vi "DSF Configuration File to Cluster.vi"(8 "error in (no error)":errorcluster, 11 "dsf configuration file path":path) -> (0 "error out":errorcluster, 2 "framework configuration out":T1, 3 "dsf configuration file path dup":path)   [LabVIEW 2017, in "DSF Core.lvlib"]
uses:
  DSF Core.lvlib
  Configuration Session.lvclass
  Read Settings.vi
  Read Plugin.vi
  Typedefs/DSF Engine Channel Configuration.ctl
  Typedefs/DSF Engine Transfer Configuration.ctl
  Typedefs/DSF Engine Transfer Group Configuration.ctl
  Typedefs/DSF Engine Plugin Configuration.ctl
  Typedefs/DSF Engine Framework Configuration.ctl
  Typedefs/DSF Settings Info.ctl
  Typedefs/DSF Timing Info.ctl
  Typedefs/DSF Byte Order.ctl
  Typedefs/DSF Data Type.ctl
  Typedefs/DSF Direction.ctl
  Read All Plugin IDs.vi
  Read Group.vi
  Typedefs/DSF Engine Plugin Thread Configuration.ctl
  Typedefs/DSF Timeout Behavior.ctl
  Read Channel.vi
  Read Transfer.vi
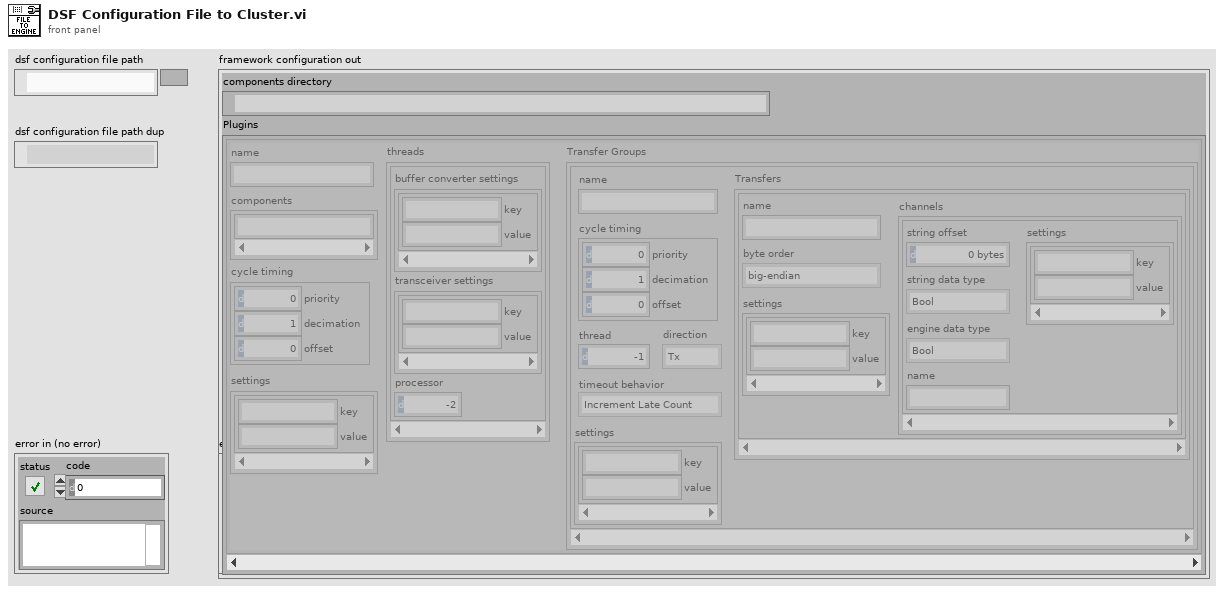
[diagram p1: front panel]
types:
  T1 = typedef "DSF Core.lvlib/DSF Engine Framework Configuration.ctl" = cluster{"components directory":path, "Plugins":T2[]}
  T2 = typedef "DSF Core.lvlib/DSF Engine Plugin Configuration.ctl" = cluster{"name":string, "components":string[], "cycle timing":T3, "threads":T4[], "Transfer Groups":T6[], "settings":T5}
  T3 = typedef "DSF Core.lvlib/DSF Timing Info.ctl" = cluster{"priority":u64, "decimation":u64, "offset":u64}
  T4 = typedef "DSF Core.lvlib/DSF Engine Plugin Thread Configuration.ctl" = cluster{"buffer converter settings":T5, "transceiver settings":T5, "processor":i32}
  T5 = typedef "DSF Core.lvlib/DSF Settings Info.ctl" = cluster{"key":string, "value":string}[]
  T6 = typedef "DSF Core.lvlib/DSF Engine Transfer Group Configuration.ctl" = cluster{"name":string, "direction":T7, "cycle timing":T3, "thread":i32, "settings":T5, "Transfers":T8[], "timeout behavior":T12}
  T7 = typedef "DSF Core.lvlib/DSF Direction.ctl" = enum8{"Tx", "Rx"}
  T8 = typedef "DSF Core.lvlib/DSF Engine Transfer Configuration.ctl" = cluster{"name":string, "byte order":T9, "settings":T5, "channels":T10[]}
  T9 = typedef "DSF Core.lvlib/DSF Byte Order.ctl" = enum8{"big-endian", "little-endian"}
  T10 = typedef "DSF Core.lvlib/DSF Engine Channel Configuration.ctl" = cluster{"string offset":u64, "string data type":T11, "engine data type":T11, "name":string, "settings":T5}
  T11 = typedef "DSF Core.lvlib/DSF Data Type.ctl" = enum8{"Bool", "SGL", "DBL", "I8", "I16", "I32", "I64", "U8", "U16", "U32", "U64"}
  T12 = typedef "DSF Core.lvlib/DSF Timeout Behavior.ctl" = enum8{"Increment Late Count", "Throw Error"}
  T13 = typedef "DSF Core.lvlib/DSF Plugin Info.ctl" = cluster{"components":string[], "timing":T3, "group ids":string[], "settings id":string, "threads":T4[]}
  T14 = typedef "DSF Core.lvlib/DSF Group Info.ctl" = cluster{"direction":T7, "timing":T3, "transfer ids":string[], "settings id":string, "thread":i32, "timeout behavior":T12}
  T15 = typedef "DSF Core.lvlib/DSF Transfer Info.ctl" = cluster{"byte order":T9, "channel ids":string[], "settings id":string}
  T16 = typedef "DSF Core.lvlib/DSF Channel Info.ctl" = cluster{"string buffer offset":u64, "string data type":T11, "engine data type":T11, "settings id":string}
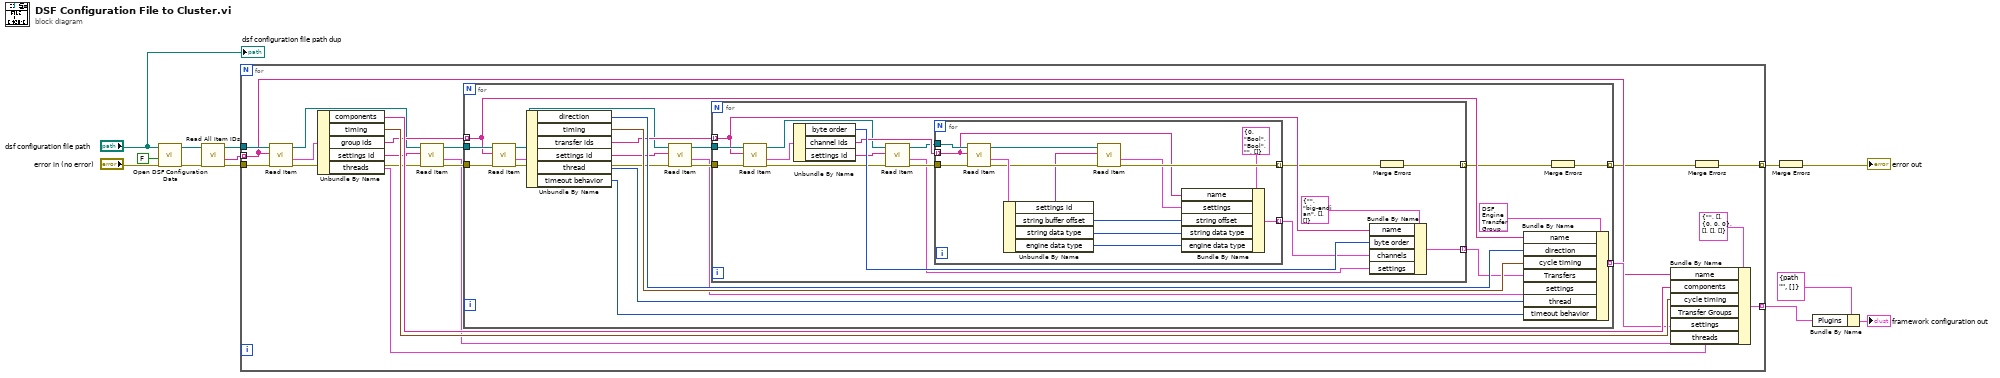
[diagram p0: block diagram]
diagram:
  n1 = call "Open DSF Configuration Data.vi"("error in (no error)"="error in (no error)", "replace if found? (F)"=FALSE ("create file if necessary (T)"), "dsf configuration file path"="dsf configuration file path") -> ("error out"=w4:errorcluster, "Configuration Session"=w5:refnum<class "Configuration Session.lvclass">)  [unwired: 4 in, 3 out]
  n2 = call-poly "Read All Item IDs.vi"("error in (no error)"=w4, "Configuration Session in"=w5) -> ("error out"=w10:errorcluster, "Plugin IDs"=w12:string[], "Configuration Session out"=w11:refnum<class "Configuration Session.lvclass">)  [unwired: 7 in]
  n3 = for {
    tunnel: w12 -> [w24] mode=indexing
    tunnel: w11 -> [w31]
    tunnel: [w27] -> w6 mode=indexing
    tunnel: w10 -> [w19]
    tunnel: [w16] -> w9 mode=indexing
    n4 = call-poly "Read Item.vi"("error in (no error)"=w19, "Plugin ID"=w24, "Configuration Session in"=w31) -> ("error out"=w20:errorcluster, "value"=w30:T13, "Configuration Session out"=w23:refnum<class "Configuration Session.lvclass">)  [unwired: 5 in, 1 out]
    n5 = Unbundle By Name(w30) -> ("components"=w29:string[], "timing"=w28:T3, "group ids"=w26:string[], "settings id"=w21:string, "threads"=w15:T4[])
    n6 = call-poly "Read Item.vi"("error in (no error)"=w20, "Settings ID"=w21, "Configuration Session in"=w23) -> ("error out"=w18:errorcluster, "value"=w14:T5, "Configuration Session out"=w22:refnum<class "Configuration Session.lvclass">)  [unwired: 5 in, 1 out]
    n7 = for {
      tunnel: w22 -> [w52]
      tunnel: w26 -> [w49] mode=indexing
      tunnel: [w46] -> w25 mode=indexing
      tunnel: w18 -> [w43]
      tunnel: [w35] -> w17 mode=indexing
      n8 = call-poly "Read Item.vi"("error in (no error)"=w43, "Group ID"=w49, "Configuration Session in"=w52) -> ("error out"=w39:errorcluster, "value"=w50:T14, "Configuration Session out"=w42:refnum<class "Configuration Session.lvclass">)  [unwired: 5 in, 1 out]
      n9 = Unbundle By Name(w50) -> ("direction"=w48:T7, "timing"=w47:T3, "transfer ids"=w45:string[], "settings id"=w40:string, "thread"=w34:i32, "timeout behavior"=w33:T12)
      n10 = call-poly "Read Item.vi"("error in (no error)"=w39, "Settings ID"=w40, "Configuration Session in"=w42) -> ("error out"=w38:errorcluster, "value"=w37:T5, "Configuration Session out"=w41:refnum<class "Configuration Session.lvclass">)  [unwired: 5 in, 1 out]
      n11 = for {
        tunnel: w45 -> [w62] mode=indexing
        tunnel: w41 -> [w69]
        tunnel: [w66] -> w44 mode=indexing
        tunnel: w38 -> [w61]
        tunnel: [w54] -> w36 mode=indexing
        n12 = call-poly "Read Item.vi"("error in (no error)"=w61, "Transfer ID"=w62, "Configuration Session in"=w69) -> ("error out"=w59:errorcluster, "value"=w68:T15, "Configuration Session out"=w63:refnum<class "Configuration Session.lvclass">)  [unwired: 5 in, 1 out]
        n13 = Unbundle By Name(w68) -> ("byte order"=w67:T9, "channel ids"=w64:string[], "settings id"=w58:string)
        n14 = call-poly "Read Item.vi"("error in (no error)"=w59, "Settings ID"=w58, "Configuration Session in"=w63) -> ("error out"=w57:errorcluster, "value"=w56:T5, "Configuration Session out"=w60:refnum<class "Configuration Session.lvclass">)  [unwired: 5 in, 1 out]
        n15 = for {
          tunnel: [w83] -> w65 mode=indexing
          tunnel: w64 -> [w74] mode=indexing
          tunnel: w60 -> [w82]
          tunnel: w57 -> [w80]
          tunnel: [w77] -> w55 mode=indexing
          n16 = call-poly "Read Item.vi"("error in (no error)"=w80, "Channel ID"=w74, "Configuration Session in"=w82) -> ("error out"=w78:errorcluster, "value"=w81:T16, "Configuration Session out"=w79:refnum<class "Configuration Session.lvclass">)  [unwired: 5 in, 1 out]
          n17 = Unbundle By Name(w81) -> ("settings id"=w75:string, "string buffer offset"=w70:u64, "string data type"=w71:T11, "engine data type"=w72:T11)
          n18 = call-poly "Read Item.vi"("error in (no error)"=w78, "Settings ID"=w75, "Configuration Session in"=w79) -> ("error out"=w77:errorcluster, "value"=w73:T5)  [unwired: 5 in, 2 out]
          n19 = Bundle By Name(cluster=T10 {"string offset"=0, "string data type"=enum."Bool", "engine data type"=enum."Bool", "name"="", "settings"=[]} ("channel configurations"), "name"=w74, "settings"=w73, "string offset"=w70, "string data type"=w71, "engine data type"=w72) -> (w83:T10)
        }
        n20 = Bundle By Name(cluster=T8 {"name"="", "byte order"=enum."big-endian", "settings"=[], "channels"=[]} ("Transfer Configuration"), "name"=w62, "byte order"=w67, "channels"=w65, "settings"=w56) -> (w66:T8)
        n21 = Merge Errors(w55) -> (w54:errorcluster)
      }
      n22 = Bundle By Name(cluster=T6 {"name"="", "direction"=enum."Tx", "cycle timing"={"priority"=0, "decimation"=0, "offset"=0}, "thread"=0, "settings"=[], "Transfers"=[], "timeout behavior"=enum."Increment Late Count"} ("Transfer Group Configuration"), "name"=w49, "direction"=w48, "cycle timing"=w47, "Transfers"=w44, "settings"=w37, "thread"=w34, "timeout behavior"=w33) -> (w46:T6)
      n23 = Merge Errors(w36) -> (w35:errorcluster)
    }
    n24 = Bundle By Name(cluster=T2 {"name"="", "components"=[], "cycle timing"={"priority"=0, "decimation"=0, "offset"=0}, "threads"=[], "Transfer Groups"=[], "settings"=[]} ("Plugin Configuration"), "name"=w24, "components"=w29, "cycle timing"=w28, "Transfer Groups"=w25, "settings"=w14, "threads"=w15) -> (w27:T2)
    n25 = Merge Errors(w17) -> (w16:errorcluster)
  }
  n26 = Merge Errors(w9) -> (→"error out":errorcluster)
  n27 = Bundle By Name(cluster=T1 {"components directory"=path "", "Plugins"=[]} ("Framework Config (JSON)"), "Plugins"=w6) -> (→"framework configuration out":T1)
  "dsf configuration file path dup" <- "dsf configuration file path"
